vi "array&graph.vi"() -> ()   [LabVIEW 2009]
panel:
  out "Waveform Chart":dbl[][](graph)
  out "Waveform Graph":dbl[][](graph)
  out "Array":dbl[][](array[numeric])
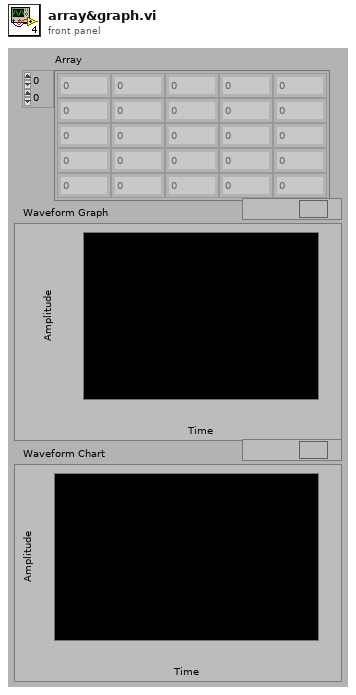
[diagram p1: front panel]
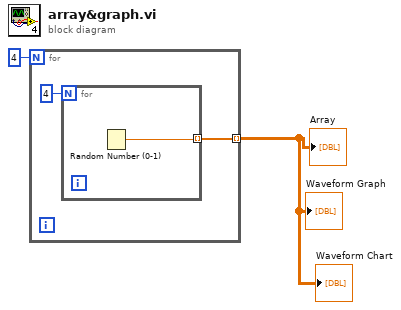
[diagram p0: block diagram]
diagram:
  n1 = for {
    N: 4 -> [_]
    tunnel: [w3] -> w1 mode=indexing
    n2 = for {
      N: 4 -> [_]
      tunnel: [w5] -> w3 mode=indexing
      n3 = Random Number (0-1)() -> (number: 0 to 1=w5:dbl)
    }
  }
  "Array" <- w1
  "Waveform Graph" <- w1
  "Waveform Chart" <- w1
